vi "Gaussian Peak Fit Coefficients (Bisquare).vi"(0 "Y":dbl[](array[numeric]), 5 "X":dbl[](array[numeric]), 7 "Weight":dbl[](array[numeric]), 9 "tolerance":dbl=-1.0 format="%#_3g", 11 "Initial Coefficients":dbl[](array[numeric])) -> (4 "amplitude":dbl, 6 "center":dbl, 8 "width":dbl, 15 "error":i32)   [LabVIEW 2017, in "NI_AALPro.lvlib"]
uses:
  <vilib>/Analysis/NI_AALPro.lvlib
  <resource>/lvanlys.dll
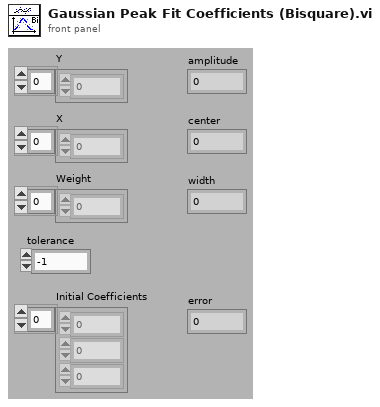
[diagram p1: front panel]
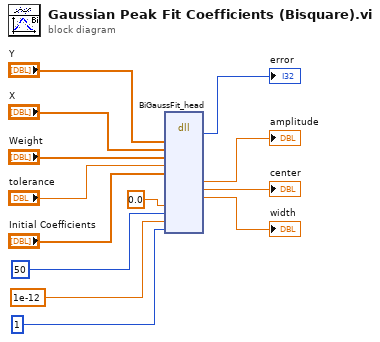
[diagram p0: block diagram]
diagram:
  n1 = dll-call lib="e:/builds/penguin/labview/branches/2017/dev/dist/resource/lvanlys.*" fn="BiGaussFit_head"("y"="Y", "x"="X", "weight"="Weight", "tolerance"="tolerance", "initialCoef"="Initial Coefficients", "meanErr"=0.0, "maxIter"=50, "absTol"=1e-12, "isCoef"=1) -> (→"error":i32, "amp"=→"amplitude":dbl, "center"=→"center":dbl, "width"=→"width":dbl)  [unwired: 15 in, 2 out]
